vi "LiftBlock.vi"   [LabVIEW 2016, in "Moving Motor.lvrbt"]
uses:
  Moving Motor.lvrbt
  <vilib>/NXT/Hardware/Plugins/Tetrix 180 deg Servo/Tetrix180ServoAddress.ctl
  <vilib>/NXT/NXTIO Xnodes/NXTIONodeSubVIs/TETRIX IO Move Servos.vi
  <vilib>/NXT/Dual Mode Library/Waits/Wait_Num.vi
  <vilib>/NXT/Subs/LVHSConnector.ctl
  <vilib>/NXT/NXTIO Xnodes/AddressXNode/NXTIOAddress.xnode
  <vilib>/NXT/NXTIO Xnodes/NXTIOXNode/NXTIO.xnode
  <vilib>/NXT/LegoClasses/BrickReference/BrickReference.lvclass
types:
  T1 = typedef "Tetrix180ServoAddress.ctl" = i32
  T2 = cluster{"Tetrix180Servo":T1, "Tetrix180Servo":T1}
  T3 = typedef "LVHSConnector.ctl" = refnum<class "BrickReference.lvclass">
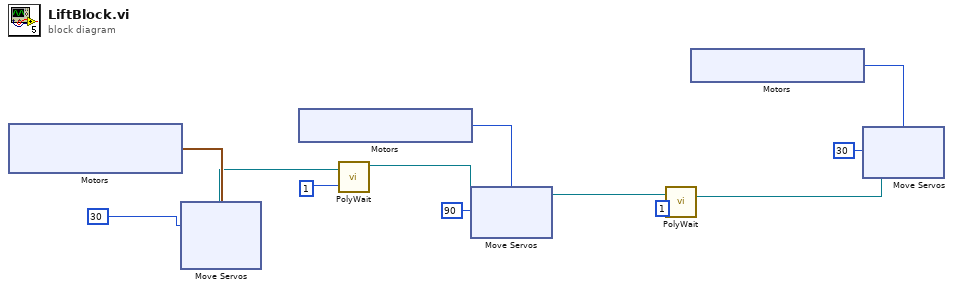
[diagram p0: block diagram]
diagram:
  n1 = xnode "Motors"() -> ("Motor"=w12:T2)
  n2 = xnode "Move Servos"("Position 1"=30, "Motors"=w12) -> ("NXT/EV3"=w8:T3)  [unwired: 2 in]
  n3 = xnode "Motors"() -> ("Motor"=w10:T1)
  n4 = call-poly <vilib>:"PolyWait.vi"("Time (1 sec)"=1, "NXT/EV3"=w8) -> ("NXT/EV3"=w6:T3)  [unwired: 2 in]
  n5 = xnode "Move Servos"("Position 1"=90, "Motors"=w10, "NXT/EV3"=w6) -> ("NXT/EV3"=w4:T3)
  n6 = call-poly <vilib>:"PolyWait.vi"("Time (1 sec)"=1, "NXT/EV3"=w4) -> ("NXT/EV3"=w1:T3)  [unwired: 2 in]
  n7 = xnode "Motors"() -> ("Motor"=w3:T1)
  n8 = xnode "Move Servos"("Position 1"=30, "Motors"=w3, "NXT/EV3"=w1) -> ()  [unwired: 1 out]
